vi "moveArc.vi"(0 "MultiAxisController in":refnum<class "_MultiAxisController.lvclass">, 1 "x_coord":i32, 2 "y_coord":i32, 3 "direction":T1, 5 "error in (no error)":errorcluster, 7 "absolute_angle (degrees)":dbl, 9 "relative_angle (degrees)":dbl) -> (14 "MultiAxisController out":refnum<class "_MultiAxisController.lvclass">, 17 "success?":bool, 18 "response":string, 19 "error out":errorcluster)   [LabVIEW 2020, in "classes.lvlib" / "_MultiAxisController.lvclass"]
doc: "Produced By:\n\n<B>Kod Integrations, LLC</B>\n4835 Marianne Drive\nMount Airy, MD 21771\nhttp://www.kodintegrations.com\nemail: info@kodintegrations.com\nphone: (240) 687-1288"
uses:
  _MultiAxisController.lvclass
  _Controller.lvclass
  C:/GEECS/Developers Version/source/Device Drivers/Newmark-NSC-A/Arcus Driver 3.0.0/ArcusUsbComm/classes/Controller/_Controller.lvclass
  C:/GEECS/Developers Version/source/Device Drivers/Newmark-NSC-A/Arcus Driver 3.0.0/ArcusUsbComm/classes/MultiAxisController/_MultiAxisController.lvclass
  circular_direction.ctl
  common.lvlib
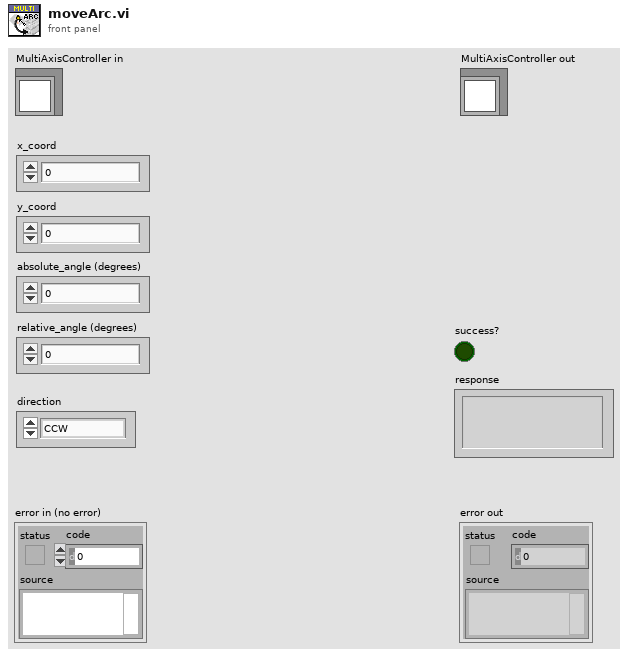
[diagram p1: front panel]
types:
  T1 = typedef "common.lvlib/circular_direction.ctl" = enum16{"CCW", "CW"}
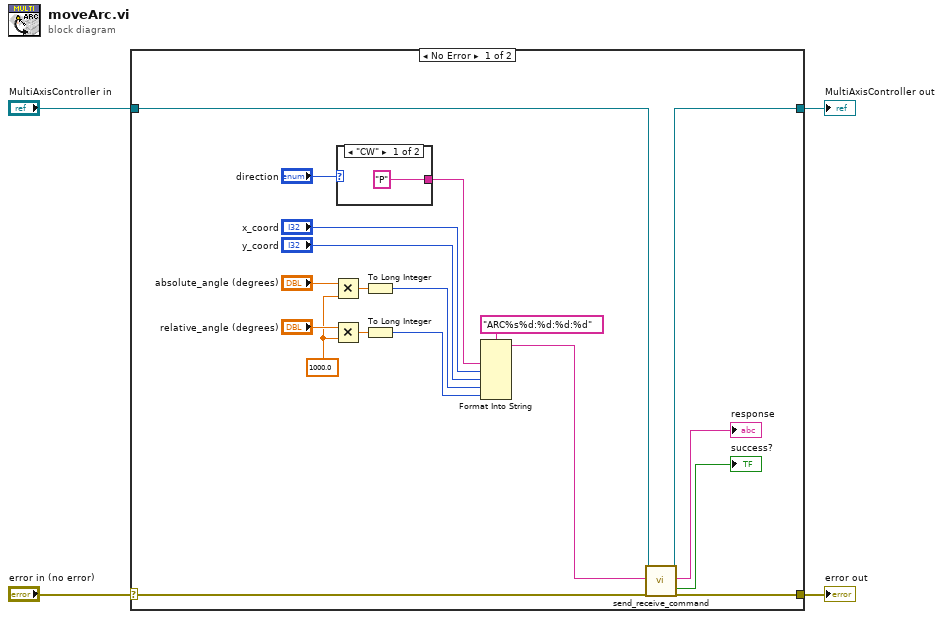
[diagram p0: block diagram]
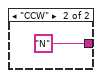
[diagram p2: hidden frame]
diagram:
  n1 = case shown="No Error" "error in (no error)" {
    selector: "error in (no error)" -> [w11 w27]
    tunnel: [w10 w27] -> w3
    tunnel: [w7 w26] -> w1
    tunnel: "MultiAxisController in" -> [w8 w26]
    frame No Error {
      w16 = 1000.0 ("y")
      n2 = Multiply(x="absolute_angle (degrees)", y=w16) -> (x*y=w15:dbl)
      n3 = Multiply(x="relative_angle (degrees)", y=w16) -> (x*y=w14:dbl)
      n4 = case shown="\"CW\"" "direction" {
        tunnel: ["P" "N"] -> w22
        frame "CW" {
        }
        frame "CCW" {
        }
      }
      n5 = To Long Integer(number=w15) -> (32bit integer=w13:i32)
      n6 = To Long Integer(number=w14) -> (32bit integer=w12:i32)
      n7 = Format Into String(format string="ARC%s%d:%d:%d:%d", w22, "x_coord", "y_coord", w13, w12) -> (resulting string=w9:string)  [unwired: 2 in, 1 out]
      n8 = call "send_receive_command.vi"("reference (in)"=w8, "ASCII Command (in)"=w9, "error in (no error)"=w11) -> ("reference (out)"=w7:refnum<class "_MultiAxisController.lvclass">, "response (out)"=→"response":string, "success?"=→"success?":bool, "error out"=w10:errorcluster)  [unwired: 12 in, 1 out]
    }
    frame Error {
    }
  }
  "error out" <- w3
  "MultiAxisController out" <- w1
